vi "T257P_Open_Port.vi"(8 "error in (no error)":errorcluster, 11 "ThermoTek T257P Port":refnum<visa-resource-name>="COM11") -> (0 "error out":errorcluster, 3 "T257P  Port OUT":refnum<visa-resource-name>="COM11")   [LabVIEW 2020]
doc: "ThermoTek T257P Labview Driver Library. © G.Shtengel. gleb.shtengel@gmail.com"
uses:
  <vilib>/Instr/_visa.llb/VISA Configure Serial Port (Instr).vi
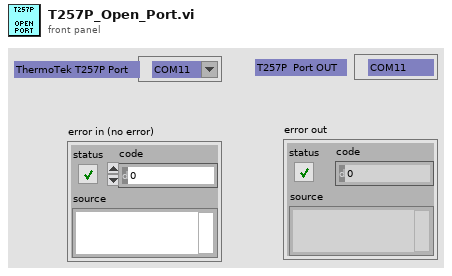
[diagram p1: front panel]
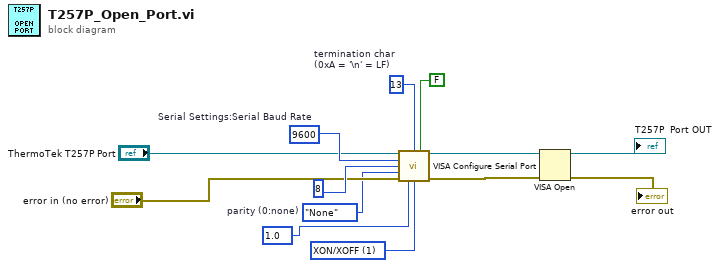
[diagram p0: block diagram]
diagram:
  w1 = u8 13  # termination char (0xA = '\n' = LF)
  w2 = enum16{"None", "Odd", "Even", "Mark", "Space"}."None"  # parity (0:none)
  w11 = u16 1 items=["None", "XON/XOFF", "RTS/CTS", "XON/XOFF & RTS/CTS", "DTR/DSR", "XON/XOFF & DTR/DSR"] ("flow control (0:none)")
  w10 = u32 9600  # Serial Settings:Serial Baud Rate
  w8 = u16 10 items=["1.0"=10, "1.5"=15, "2.0"=20] ("Serial Settings:Serial Stop Bits")
  n1 = call-poly "VISA Configure Serial Port"("VISA resource name"="ThermoTek T257P Port", "termination char\n(0xA = '\\n' = LF)"=w1, "Enable Termination\nChar (T)"=FALSE ("Message Based Settings:Termination Character Enable"), "baud rate (9600)"=w10, "data bits (8)"=u16 8 ("Serial Settings:Serial Data Bits"), "parity (0:none)"=w2, "error in (no error)"="error in (no error)", "stop bits (10: 1 bit)"=w8, "flow control (0:none)"=w11) -> ("VISA resource name out"=w4:refnum<visa-resource-name>, "error out"=w3:errorcluster)  [unwired: 5 in]
  n2 = VISA Open(error in (no error)=w3, VISA resource name=w4) -> (VISA resource name=→"T257P  Port OUT":refnum<visa-resource-name>, error out=→"error out":errorcluster)  [unwired: 3 in]
